vi "OpenDeviceMSOOnly.vi"(0 "object in":refnum<class "AD2_MSO_SDK.lvclass">, 5 "error in (no error)":errorcluster) -> (14 "object out":refnum<class "AD2_MSO_SDK.lvclass">, 19 "error out":errorcluster)   [LabVIEW 2019, in "AD2_MSO_SDK.lvclass"]
uses:
  AD2_MSO_SDK.lvclass
  AD2_MSO_SDK.lvclass/AD2_MSO_SDK.ctl
  Olasdwf/Olasdwf.lvlib
panel:
  out "AD2DeviceName":string
  out "AD2Serial":string
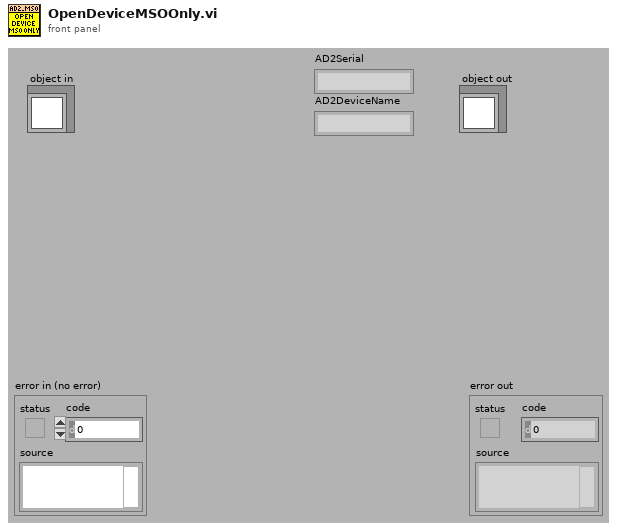
[diagram p1: front panel]
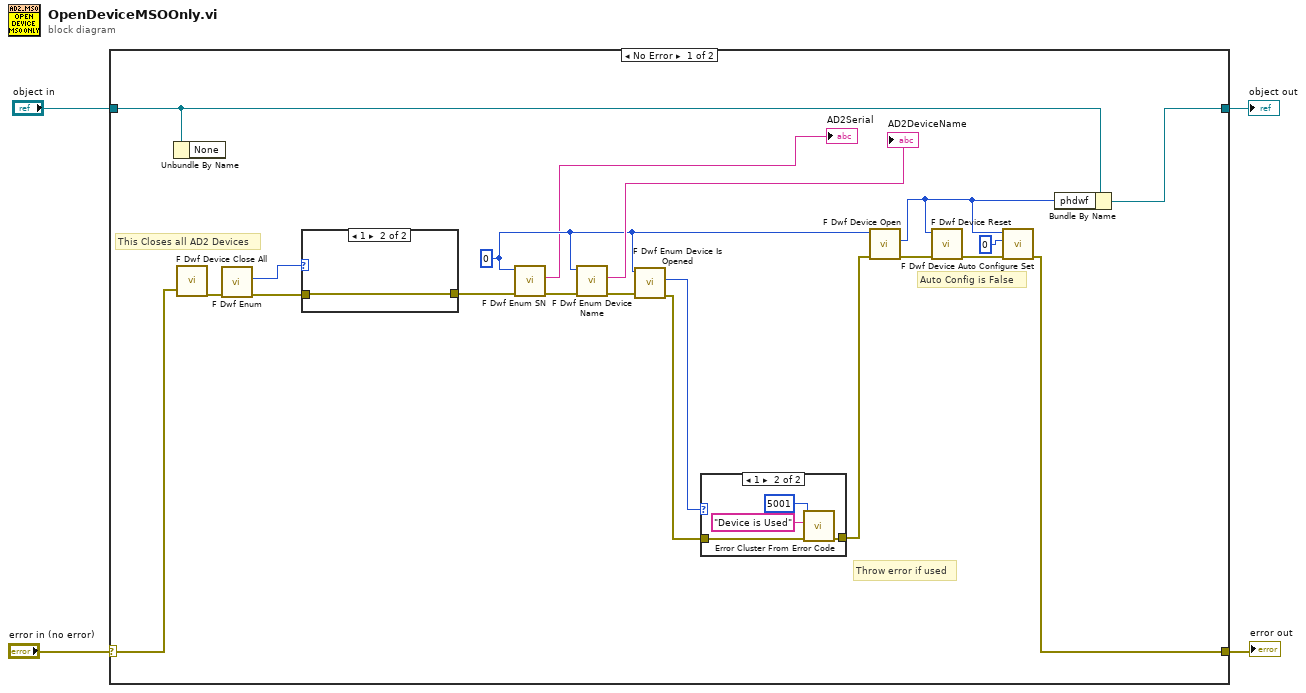
[diagram p0: block diagram]
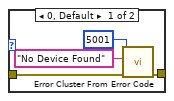
[diagram p3: hidden frame]
diagram:
  n1 = case shown="No Error" "error in (no error)" {
    selector: "error in (no error)" -> [w8 w36]
    tunnel: [w7 w36] -> w3
    tunnel: [w6 w35] -> w1
    tunnel: "object in" -> [w5 w35]
    frame No Error {
      w13 = 0 ("idxDevice")
      # "Auto Config is False"
      # "This Closes all AD2 Devices"
      # "Throw error if used"
      n2 = Unbundle By Name(w5) -> ()  [unwired: 1 out]
      n3 = call "F Dwf Device Close All.vi"("error in (no error)"=w8) -> ("error out"=w22:errorcluster)  [unwired: 9 in, 1 out]
      n4 = call "F Dwf Enum.vi"("error in (no error)"=w22) -> ("error out"=w10:errorcluster, "pcDevice out"=w11:i32)  [unwired: 8 in, 1 out]
      n5 = case shown="1" w11 {
        tunnel: w10 -> [w32 w34]
        tunnel: [w31 w34] -> w9
        frame 0, Default {
          n6 = call <vilib>:"Error Cluster From Error Code.vi"("error in (no error)"=w32, "error message (\"\")"="No Device Found" ("error message (\"\")"), "error code (0)"=5001) -> ("error out"=w31:errorcluster)  [unwired: 6 in]
        }
        frame 1 {
        }
      }
      n7 = call "F Dwf Enum SN.vi"("error in (no error)"=w9, "idxDevice"=w13) -> ("error out"=w24:errorcluster, "szSN out"=→"AD2Serial":string)  [unwired: 7 in, 1 out]
      n8 = call "F Dwf Enum Device Name.vi"("error in (no error)"=w24, "idxDevice"=w13) -> ("error out"=w16:errorcluster, "szDeviceName out"=→"AD2DeviceName":string)  [unwired: 7 in, 1 out]
      n9 = call "F Dwf Enum Device Is Opened.vi"("error in (no error)"=w16, "idxDevice"=w13) -> ("error out"=w15:errorcluster, "pfIsUsed out"=w14:i32)  [unwired: 7 in, 1 out]
      n10 = case shown="1" w14 {
        tunnel: w15 -> [w25 w28]
        tunnel: [w25 w27] -> w17
        frame 0, Default {
        }
        frame 1 {
          n11 = call <vilib>:"Error Cluster From Error Code.vi"("error in (no error)"=w28, "error message (\"\")"="Device is Used" ("error message (\"\")"), "error code (0)"=5001) -> ("error out"=w27:errorcluster)  [unwired: 6 in]
        }
      }
      n12 = call "F Dwf Device Open.vi"("error in (no error)"=w17, "idxDevice"=w13) -> ("error out"=w21:errorcluster, "phdwf out"=w18:i32)  [unwired: 7 in, 1 out]
      n13 = call "F Dwf Device Reset.vi"("error in (no error)"=w21, "hdwf"=w18) -> ("error out"=w20:errorcluster)  [unwired: 8 in, 1 out]
      n14 = call "F Dwf Device Auto Configure Set.vi"("error in (no error)"=w20, "fAutoConfigure"=0, "hdwf"=w18) -> ("error out"=w7:errorcluster)  [unwired: 7 in, 1 out]
      n15 = Bundle By Name(cluster=w5, "phdwf"=w18) -> (w6:refnum<class "AD2_MSO_SDK.lvclass">)
    }
    frame Error {
    }
  }
  "error out" <- w3
  "object out" <- w1
